vi "dfd_Apply Window.vi"(8 "error in (no error)":errorcluster, 9 "window param":dbl, 10 "window":u16(ring)=1 items=["None"=0, "Hanning"=1, "Hamming"=2, "Blackman-Harris"=3, "Exact Blackman"=4, "Blackman"=5, "Flat Top"=6, "4 Term B-Harris"=7, "7 Term B-Harris"=8, "Low Sidelobe"=9, "Triangular"=30, "Kaiser"=60, "Dolph-Chebyshev"=61, "Gaussian"=62], 11 "x":dbl[](array[numeric]) format="%.2f") -> (0 "error out":errorcluster, 3 "windowed x":dbl[](array[numeric]))   [LabVIEW 2017, in "NI_DigFilter_Design.lvlib"]
uses:
  <vilib>/addons/Digital Filter Design/NI_DigFilter_Design.lvlib
  <vilib>/addons/Digital Filter Design/_Misc.llb/dfd_Error Cluster From Error Code (Scalar).vi
  <vilib>/Analysis/0measdsp.llb/Scaled Time Domain Window (DBL).vi
  <vilib>/addons/Digital Filter Design/NI_DigFilterLicensed.lvlib
  <vilib>/Analysis/NI_AALPro.lvlib
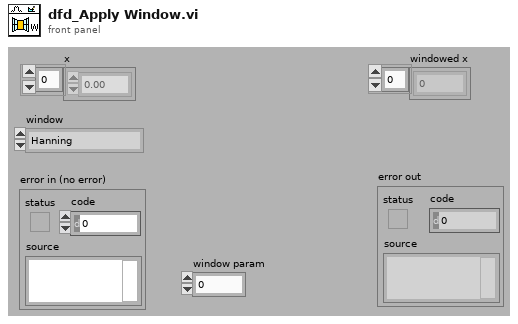
[diagram p1: front panel]
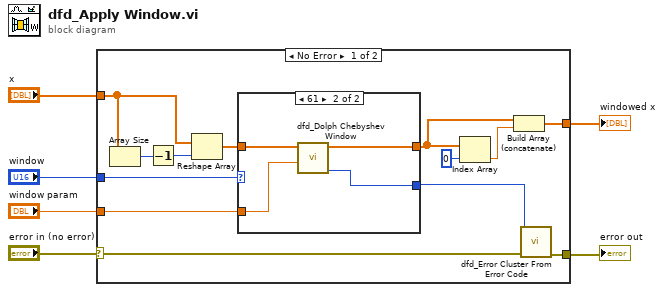
[diagram p0: block diagram]
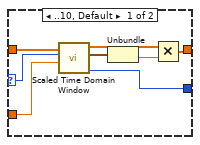
[diagram p2: hidden frame]
diagram:
  n1 = case shown="No Error" "error in (no error)" {
    selector: "error in (no error)" -> [w16 w32]
    tunnel: "window" -> [w10 _]
    tunnel: [w17 w32] -> w5
    tunnel: "x" -> [w14 _]
    tunnel: [w12 _] -> w4
    tunnel: "window param" -> [w9 _]
    frame No Error {
      n2 = Array Size(array=w14) -> (size(s)=w15:i32)
      n3 = Decrement(x=w15) -> (x-1=w13:i32)
      n4 = Reshape Array(w14, w13) -> (w11:dbl[])
      n5 = case shown="61" w10 {
        selector: w10 -> [w22 _]
        tunnel: [w24 w30] -> w8
        tunnel: w11 -> [w27 w31]
        tunnel: [w20 w28] -> w7
        tunnel: w9 -> [w21 w29]
        frame ..10, Default {
          n6 = call-poly <vilib>:"Scaled Time Domain Window.vi"("window parameter"=w21, "window"=w22, "X"=w27) -> ("error"=w20:i32, "window properties"=w25:cluster{"eq noise BW":dbl, "coherent gain":dbl}, "Windowed X"=w26:dbl[])  [unwired: 6 out]
          n7 = Unbundle(w25) -> ("coherent gain"=w23:dbl)  [unwired: 1 out]
          n8 = Multiply(x=w26, y=w23) -> (x*y=w24:dbl[])
        }
        frame 61 {
          n9 = call <vilib>:"dfd_Dolph Chebyshev Window.vi"("r [dB]"=w29, "x(t)"=w31) -> ("error"=w28:i32, "Dolph-Chebyshev"=w30:dbl[])  [unwired: 8 out]
        }
      }
      n10 = Index Array(array=w8, index=0) -> (element=w19:dbl)
      n11 = Build Array (concatenate)(w8, w19) -> (w12:dbl[])
      n12 = call-poly <vilib>:"dfd_Error Cluster From Error Code.vi"("error in (no error)"=w16, "error code (0)"=w7) -> ("error out"=w17:errorcluster)  [unwired: 9 out]
    }
    frame Error {
    }
  }
  "error out" <- w5
  "windowed x" <- w4
